vi "testCAN 3 tcpip.vi"() -> ()   [LabVIEW 2014]
uses:
  <vilib>/Utility/Variable/NI_VariableUtilities.lvlib
  Documents/LabVIEW Data/Untitled Project 2/support/Message Queue/Message Cluster.ctl
  Documents/LabVIEW Data/Untitled Project 2/support/Message Queue/Message Queue.lvlib
  <vilib>/Utility/inputDevices.llb/joystickAcquire.vi
  <vilib>/NI/STM/TCP/Read Message (TCP).vi
  <vilib>/NI/STM/TCP/Get Connection Reference (TCP).vi
  <vilib>/NI/STM/TCP/Read Meta Data (TCP Ref).vi
  CANFrameControl.ctl
panel:
  out "can z sb":T1 {"type" items=["CAN Data", "CAN Remote"]; "identifier" format="%.0x"}
  in  "stop 3":bool
  out "Iteration Counter":i32
  in  "Target IP Address":string="localhost"
  out "error  out":errorcluster
  out "ilosc mesag":dbl
  in  "Boolean":bool
  out "Numeric 2":i32
  in  "stop event":bool
  in  "Tab Control":T2(tab)
  in  "Przód":T3
  out "size(s)":i32[](array[numeric])
  in  "identifier 2":u32 format="%x"
  in  "identifier":u32 format="%x"
  out "Numeric":i32
  in  "stop 2":bool
  out "Ramki CAN":T1[](array[typedef]) {"type" items=["CAN Data", "CAN Remote"]; "identifier" format="%.0x"}
  in  "Adres sbRio":string
  out "output 5":u16
  out "output 4":u16
  out "element 2":string
  out "element":string
  out "output 2":u16
  out "output 3":u16
  in  "device index":i32
  in  "Number of Frames to Display":i32=15
  out "Frames":string[][](table)
  in  "stop":bool
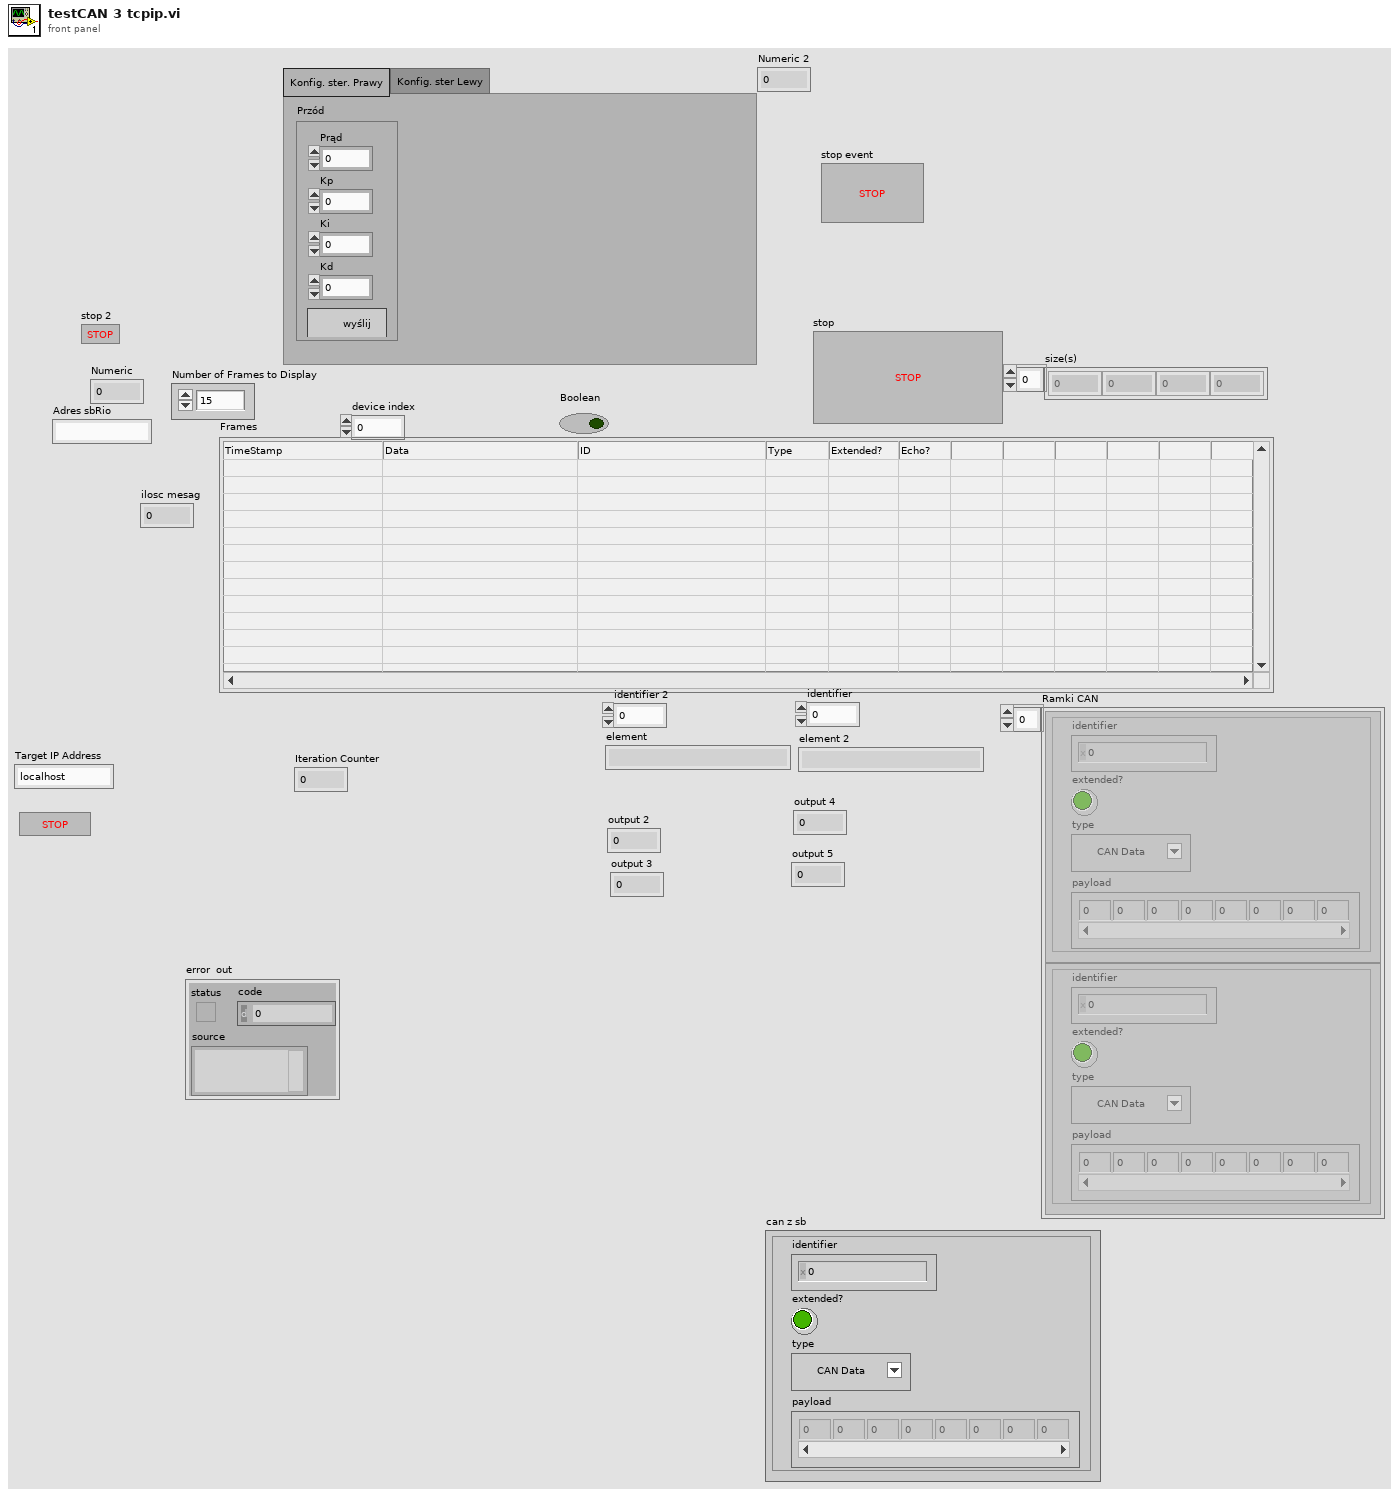
[diagram p1: front panel]
types:
  T1 = typedef "CANFrameControl.ctl" = cluster{"identifier":u32, "extended?":bool, "type":u8, "payload":u8[]}
  T2 = enum32{"Konfig. ster. Prawy", "Konfig. ster Lewy"}
  T3 = cluster{"Prąd":u16, "Kp":u16, "Ki":u16, "Kd":u16, "OK Button":bool}
  T4 = cluster{"X axis":i32, "Y axis":i32, "Z axis":i32, "X axis rotation":i32, "Y axis rotation":i32, "Z axis rotation":i32, "U axis":i32, "V axis":i32}
  T5 = cluster{"button 1":bool, "button 2":bool, "button 3":bool, "button 4":bool, "button 5":bool, "button 6":bool, "button 7":bool, "button 8":bool, "button 9":bool, "button 10":bool, "button 11":bool, "button 12":bool, "button 13":bool, "button 14":bool, "button 15":bool, "button 16":bool, "button 17":bool, "button 18":bool, "button 19":bool, "button 20":bool, "button 21":bool, "button 22":bool, "button 23":bool, "button 24":bool, "button 25":bool, "button 26":bool, "button 27":bool, "button 28":bool, "button 29":bool, "button 30":bool, "button 31":bool, "button 32":bool}
  T6 = typedef "Message Queue.lvlib/Message Cluster.ctl" = cluster{"Message":string, "Message Data":variant}
  T7 = typedef "NI STM.lvlib/TCP Connection Info.ctl" = cluster{"connection ID":refnum<k5>, "meta data":T8[]}
  T8 = typedef "NI STM.lvlib/MetaDataElement.ctl" = string
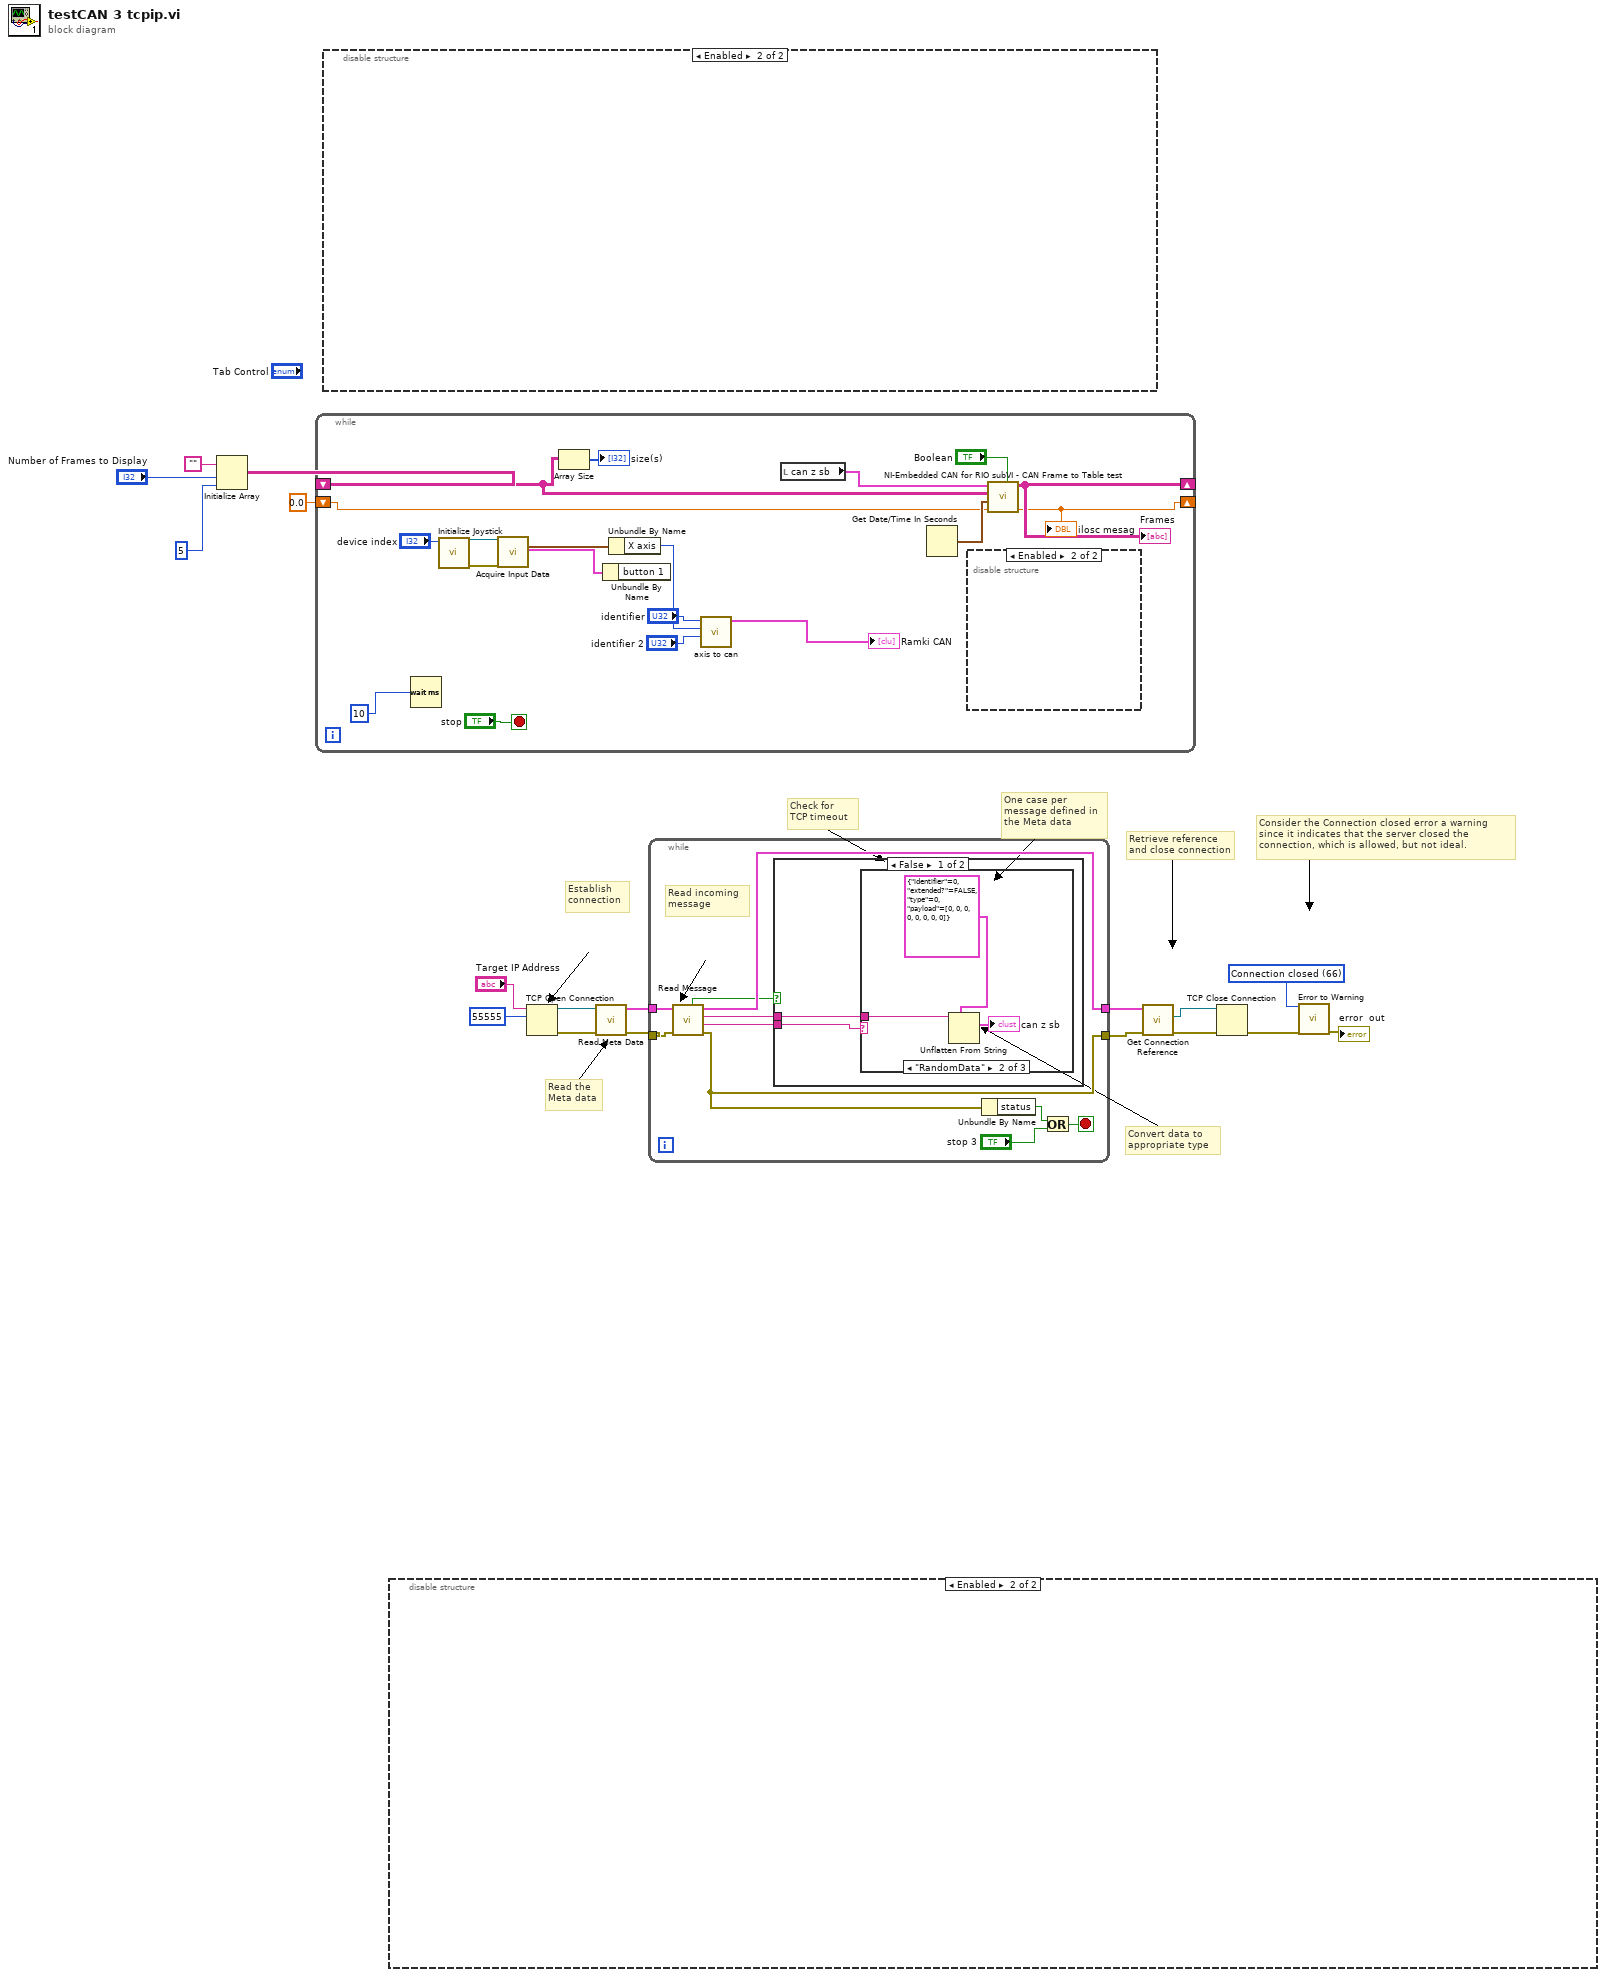
[diagram p0: block diagram]
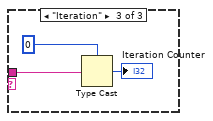
[diagram p3: hidden frame]
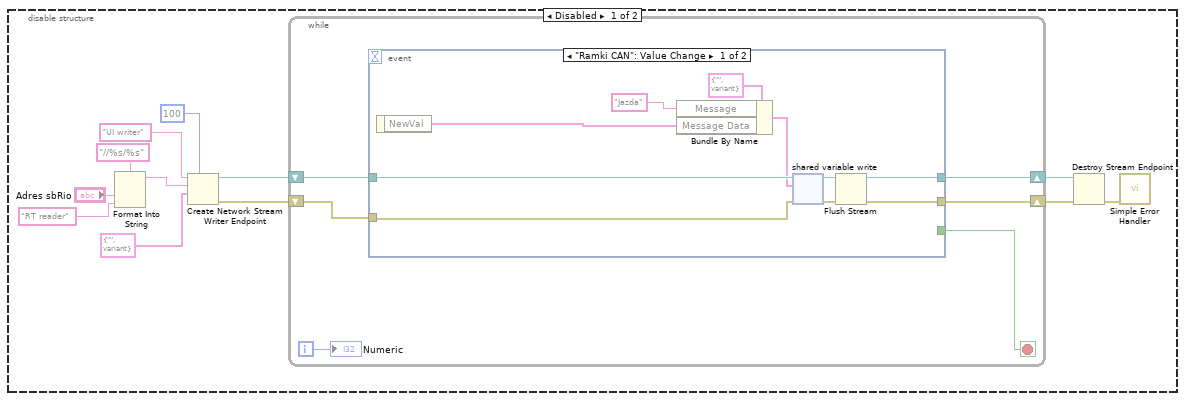
[diagram p5: hidden frame]
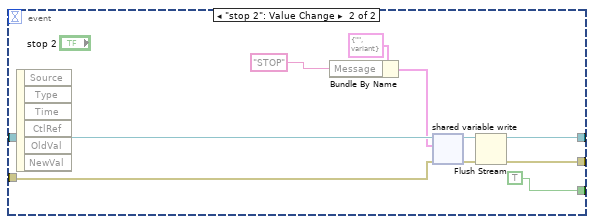
[diagram p6: hidden frame]
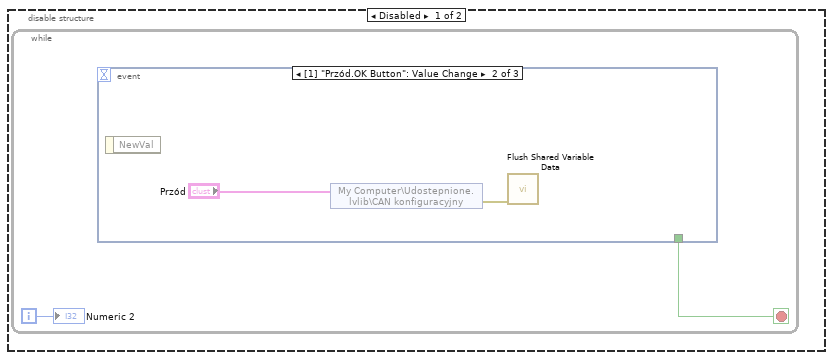
[diagram p7: hidden frame]
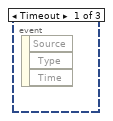
[diagram p8: hidden frame]
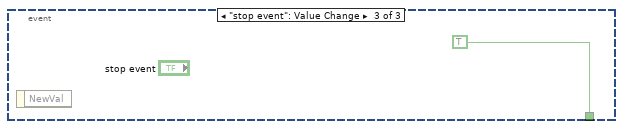
[diagram p9: hidden frame]
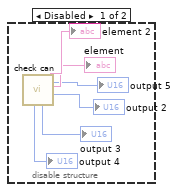
[diagram p10: hidden frame]
diagram:
  w7 = 66 items=["No Error", "Argument Error", "Memory Full", "Out of Zone", "End of File", "File Already Open", "Generic File IO Error", "File Not Found", "File Permission Error", "Disk Full", "Duplicate Path", "Too Many Files Open", "Not Enabled", "Resource File Not Found", "Cannot Add Resource", "Resource Not Found", "Image Not Found", "Image Memory Error", "Pen Does Not Exist", "Config Bad Type", "Config Token Not Found", "Config Parse Error", "Config Memory Error", "Bad External Code Format", "Bad External Code Offset", "External Code Not Present", "Null Window", "Destroy Window Mixup", "Null Menu", "Print Aborted", "Bad Print Record", "Print Driver Error", "Windows Error During Print", "Memory Error During Print", "Print Dialog Error", "Generic Print Error", "Invalid Device Refnum", "Device Not Found", "Device Parameter Error", "Device Unit Error", "Can't Open Device", "Device Call Aborted", "Generic Error", "Cancelled By User", "Object ID Too Low", "Object ID Too High", "Object Not In Heap", "Unknown Heap", "Bad DefProc ID", "DefProc Not In Table", "Message Out Of Range", "Null Method", "Unknown Message", "Manager Call Not Supported", "Bad address", "Connection In progress", "Connection timed out", "Connection is already in progress", "Network attribute not supported", "Network error", "Address in use", "System out of memory", "Connection aborted", "Connection refused", "Connection is not connected", "Connection is already connected", "Connection closed", "Initialize error (interapplication manager)", "Bad occurrence", "Wait on unbound occurrence handler", "Occurrence queue overflow", "Bad path", "Semaphore not signaled", "Unrecognized type (interapplication manager)"] ("1st Error to Convert")
  # "Consider the Connection closed error a warning since it indicates that the server closed the connection, which is allowed, but not ideal."
  # "Retrieve reference and close connection"
  # "Check for\nTCP timeout"
  # "Convert data to\nappropriate type"
  # "One case per\nmessage defined in\nthe Meta data"
  # "Read the \nMeta data"
  # "Establish\nconnection"
  n1 = Initialize Array("" ("Empty String Constant"), "Number of Frames to Display", 5 ("dimension size")) -> (w15:string[][])
  n2 = while {
    shift-right: [w23] -> _
    shift-left: w15 -> [w26]
    shift-right: [w21] -> _
    shift-left: 0.0 ("Numeric") -> [w20]
    stop <- "stop" stop-if-true
    n3 = Wait (ms)(milliseconds to wait=u32 10) -> ()  [unwired: 1 out]
    n4 = call <vilib>:"Initialize Joystick.vi"("device index"="device index") -> ("error out"=w35:errorcluster, "device ID"=w36:refnum<k1>)  [unwired: 9 in]
    n5 = call-poly <vilib>:"Acquire Input Data.vi"("device ID"=w36, "error in (no error)"=w35) -> ("axis info"=w33:T4, "button info"=w32:T5)  [unwired: 13 in, 3 out]
    n6 = Array Size(array=w26) -> (size(s)=→"size(s)":i32[])
    n7 = Unbundle By Name(w32) -> ()  [unwired: 1 out]
    n8 = Unbundle By Name(w33) -> ("X axis"=w31:i32)
    n9 = call "axis to can.vi"("wyślij"="identifier 2", "wej wagi"=w31, "wej ster"="identifier") -> ("druga ramka"=→"Ramki CAN":T1)  [unwired: 3 in, 5 out]
    n10 = local read "can z sb"() -> (w22:T1)
    n11 = Get Date/Time In Seconds() -> (seconds since 1Jan1904=w27:timestamp)
    n12 = disable-structure shown="Enabled" {
      frame Disabled {
        n13 = call "check can.vi"() -> ("Numeric"=→"output 2":u16, "element"=→"element":string, "element 2"=→"element 2":string, "output 3"=→"output 3":u16, "output 5"=→"output 5":u16, "output 4"=→"output 4":u16)  [unwired: 6 in]
      }
      frame Enabled {
      }
    }
    n14 = call "NI-Embedded CAN for RIO subVI - CAN Frame to Table test.vi"("Boolean"="Boolean", "x"=w20, "timestamp"=w27, "Input Array"=w26, "CAN frame"=w22) -> ("Numeric"=w21:dbl, "Output Array"=w23:string[][])  [unwired: 2 in, 3 out]
    "Frames" <- w23
    "ilosc mesag" <- w21
  }
  n15 = disable-structure shown="Enabled" {
    frame Disabled {
      n16 = while {
        i -> [w44]
        stop <- w45 stop-if-true
        n17 = event shown="[1] \"Przód.OK Button\": Value Change" {
          selector: _ -> [_ _ _]
          dyn-events: _ -> [_ _ _]
          timeout: _ -> [_ _ _]
          tunnel: [_ _ TRUE] -> w45
          event Timeout {
            n18 = event-data() -> ()  [unwired: 1 in, 3 out]
          }
          event "Przód.OK Button": Value Change {
            n19 = event-data() -> ()  [unwired: 1 in, 1 out]
            n20 = shared-variable "My Computer\\Udostepnione.lvlib\\CAN konfiguracyjny"("Przód") -> (error out=w46:errorcluster)  [unwired: 1 in]
            n21 = call <vilib>:"Flush Shared Variable Data.vi"("error in (no error)"=w46) -> ()  [unwired: 10 in, 1 out]
          }
          event "stop event": Value Change {
            n22 = event-data() -> ()  [unwired: 1 in, 1 out]
          }
        }
        "Numeric 2" <- w44
      }
    }
    frame Enabled {
    }
  }
  n23 = disable-structure shown="Enabled" {
    frame Disabled {
      n24 = Format Into String(format string="//%s/%s", "Adres sbRio", "RT reader" ("writer name")) -> (resulting string=w58:string)  [unwired: 2 in, 1 out]
      n25 = Create Network Stream Writer Endpoint(7:100 ("writer buffer size"), 9:T6 {"Message"="", "Message Data"=variant} ("Message Cluster"), 10:w58, 11:"UI writer" ("writer name")) -> (0:w54:errorcluster, 3:w55:refnum<k21>)  [unwired: 3 in]
      n26 = while {
        shift-right: [w65] -> w52
        shift-left: w55 -> [w66]
        shift-right: [w64] -> w51
        shift-left: w54 -> [w63]
        i -> [w61]
        stop <- w62 stop-if-true
        n27 = event shown="[0] \"Ramki CAN\": Value Change" {
          selector: _ -> [_ _]
          dyn-events: _ -> [_ _]
          timeout: _ -> [_ _]
          tunnel: w66 -> [w73 w83]
          tunnel: [w70 w80] -> w65
          tunnel: [w69 w79] -> w64
          tunnel: w63 -> [w68 w78]
          tunnel: [_ TRUE] -> w62
          event "Ramki CAN": Value Change {
            n28 = event-data() -> ("NewVal"=w67:T1[])  [unwired: 1 in]
            n29 = Bundle By Name(cluster=T6 {"Message"="", "Message Data"=variant} ("Message Cluster"), "Message"="Jazda", "Message Data"=w67) -> (w72:T6)
            n30 = shared-variable-write(w73, w68, w72) -> (w75:refnum<k21>, w76:errorcluster)  [unwired: 1 in, 1 out]
            n31 = Flush Stream(8:w76, 11:w75) -> (0:w69:errorcluster, 3:w70:refnum<k21>)  [unwired: 2 in, 1 out]
          }
          event "stop 2": Value Change {
            n32 = event-data() -> ()  [unwired: 1 in, 6 out]
            n33 = Bundle By Name(cluster=T6 {"Message"="", "Message Data"=variant} ("Message Cluster"), "Message"="STOP") -> (w82:T6)
            n34 = shared-variable-write(w83, w78, w82) -> (w85:refnum<k21>, w86:errorcluster)  [unwired: 1 in, 1 out]
            n35 = Flush Stream(8:w86, 11:w85) -> (0:w79:errorcluster, 3:w80:refnum<k21>)  [unwired: 2 in, 1 out]
          }
        }
        "Numeric" <- w61
      }
      n36 = Destroy Stream Endpoint(8:w51, 11:w52) -> (0:w53:errorcluster)
      n37 = call <vilib>:"Simple Error Handler.vi"("error in (no error)"=w53) -> ()  [unwired: 4 in, 5 out]
    }
    frame Enabled {
    }
  }
  n38 = TCP Open Connection(address="Target IP Address", remote port or service name=u16 55555 ("remote port")) -> (connection ID=w1:refnum<k5>, error out=w3:errorcluster)  [unwired: 1 in, 2 out]
  n39 = call-poly <vilib>:"Read Meta Data.vi"("error in"=w3, "connection ID"=w1) -> ("error out"=w4:errorcluster, "connection info out"=w2:T7)  [unwired: 1 in, 7 out]
  n40 = while {
    tunnel: w2 -> [w96]
    tunnel: w4 -> [w95]
    tunnel: [w94] -> w10
    tunnel: [w91] -> w11
    stop <- w88 stop-if-true
    # "Read incoming\nmessage"
    n41 = call-poly <vilib>:"Read Message.vi"("error in"=w95, "connection info in"=w96) -> ("error out"=w91:errorcluster, "name"=w93:T8, "data string"=w92:string, "connection info out"=w94:T7, "timed out?"=w87:bool)  [unwired: 1 in, 4 out]
    n42 = case shown="False" w87 {
      tunnel: w93 -> [w97 _]
      tunnel: w92 -> [w98 _]
      frame False {
        n43 = case shown="\"RandomData\"" w97 {
          tunnel: w98 -> [_ w101 w104]
          frame Default {
          }
          frame "RandomData" {
            n44 = Unflatten From String(type=T1 {"identifier"=0, "extended?"=FALSE, "type"=0, "payload"=[0, 0, 0, 0, 0, 0, 0, 0]} ("CAN frame"), binary string=w101) -> (value=→"can z sb":T1)  [unwired: 1 in, 4 out]
          }
          frame "Iteration" {
            n45 = Type Cast(type=0, x=w104) -> (*(type *) &x=→"Iteration Counter":i32)
          }
        }
      }
      frame True {
      }
    }
    n46 = Unbundle By Name(w91) -> ("status"=w90:bool)
    n47 = Or(x=w90, y="stop 3") -> (x .or. y?=w88:bool)
  }
  n48 = call-poly <vilib>:"Get Connection Reference.vi"("error in"=w11, "connection info in"=w10) -> ("error out"=w13:errorcluster, "connection ID out"=w12:refnum<k5>)  [unwired: 8 out]
  n49 = TCP Close Connection(connection ID=w12, error in (no error)=w13) -> (error out=w8:errorcluster)  [unwired: 2 out]
  n50 = call <vilib>:"Error to Warning.vi"("1st Error to Convert"=w7, "error in"=w8) -> ("warning out"=→"error  out":errorcluster)  [unwired: 3 in, 10 out]
